vi "Synchronized Acquisition with Disk Streaming.vi"() -> ()   [LabVIEW 2021]
uses:
  <vilib>/userdefined/Silver/nirio_resource_slv.ctl
  Digitizer Control Class/Public/TClk API Control Enable.ctl
  Digitizer Control Class/Digitizer Control.lvclass
  Disk Streaming Class/Disk Streaming.lvclass
  Disk Streaming Class/Public/IO mode.ctl
  Digitizer Control Class/Public/Acq Start Trigger Type.ctl
panel:
  in  "PXIe?":bool=TRUE
  out "Samples Acquired":u64[](array[numeric])
  in  "Stop Button":bool
  in  "Tab Control":enum32{"Acquisition Preview", "I/O Performance"}(tab)
  out "Waveform Graph":waveform(dbl)[](graph)
  out "Power Spectrum":cluster{"f0":dbl, "df":dbl, "magnitude":dbl[]}[](graph) caption="Waveform Graph"
  out "Pending Disk Operations":u32[](graph)
  out "Host DMA buffer use":u64[](graph)
  out "Device Memory use":u64[][](graph)
  out "Device FIFO use":u64[][](graph)
  in  "# of blocks":u32=5
  in  "Preview # of samples":u32=10000
  in  "Reserve File Size?":bool
  in  "Disable Buffering?":bool=TRUE
  in  "I/O mode":T1(ring)=enum."Data Reference"
  in  "Block Duration (s)":dbl=0.01 format="%0.2p"
  in  "12-bit packing":bool
  out "Overflow":bool[](array[boolean])
  in  "Desired Sampling Rate":dbl=800000000.0 format="%0.2p"
  out "Actual IQ Rate":dbl format="%#_6p"
  in  "# of samples":i64=10000000
  in  "device and file selection":T3(array[cluster])
  # "Device / File Selection"
  # "Device"
  # "AI0 Destination File"
  # "AI1 Destination File"
  # "Acquisition Configuration"
  # "Acquisition Status"
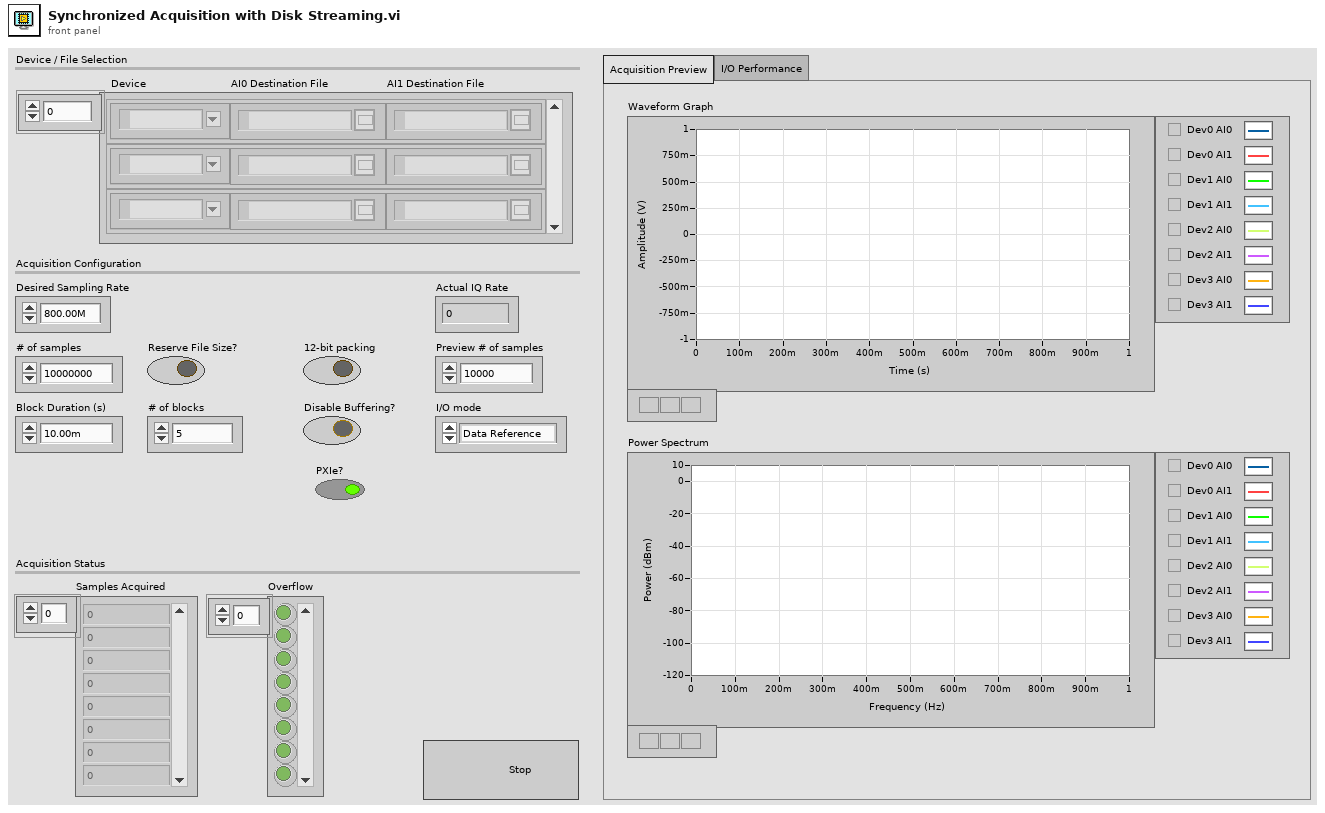
[diagram p1: front panel]
types:
  T1 = enum16{"Synchronous", "Asynchronous", "Data Reference"}
  T2 = typedef "nirio_resource_slv.ctl" = tag
  T3 = cluster{"RIO Device":T2, "AI0 File":path, "AI1 File":path}[]
  T4 = typedef "Digitizer Control.lvclass/TClk API Control Enable.ctl" = enum16{"None", "Acquisition"}
  T5 = typedef "Disk Streaming.lvclass/IO mode.ctl" = enum16{"Synchronous", "Asynchronous", "Data Reference"}
  T6 = cluster{"enabled":bool, "session":refnum<class "Digitizer Control.lvclass">, "channel index":i32, "sample count":i64, "disk streaming":refnum<class "Disk Streaming.lvclass">, "I/O mode":T5}
  T7 = typedef "Digitizer Control.lvclass/Acq Start Trigger Type.ctl" = enum16{"Immediate", "Analog", "Digital Edge", "Digital Level"}
  T8 = cluster{"enabled":bool, "session":refnum<class "Digitizer Control.lvclass">, "channel index":i32, "sample count":i64, "disk streaming":refnum<class "Disk Streaming.lvclass">, "I/O mode":T5}[]
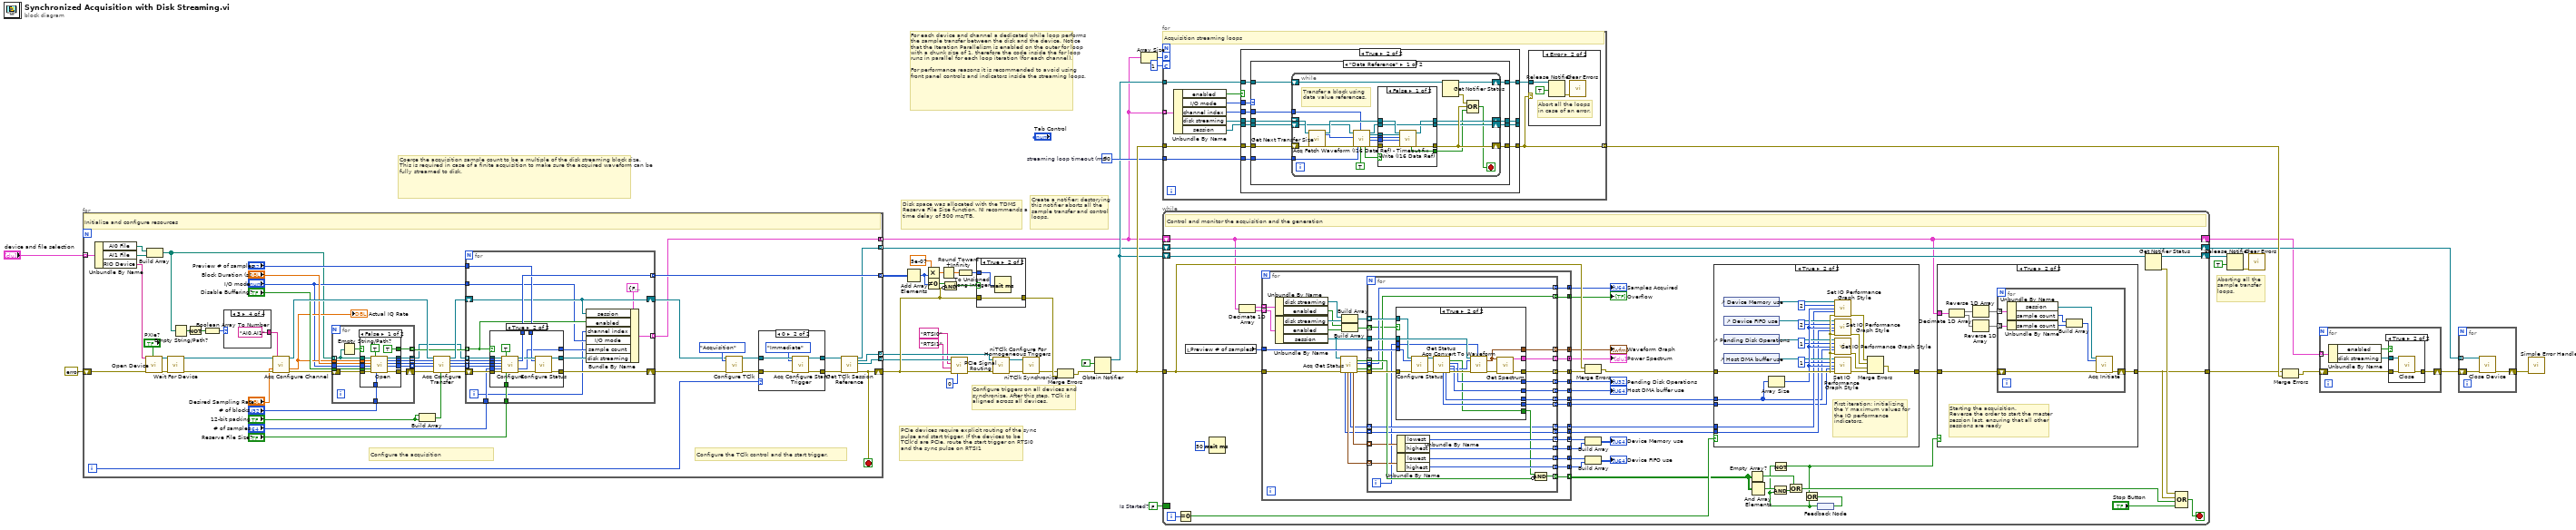
[diagram p0: block diagram]
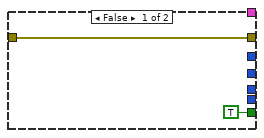
[diagram p5: hidden frame]
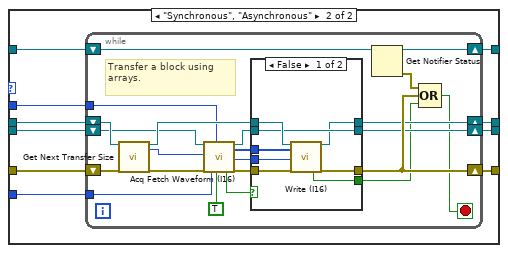
[diagram p9: hidden frame]
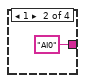
[diagram p13: hidden frame]
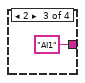
[diagram p14: hidden frame]
diagram:
  w5 = FALSE  # Is Started?
  w14 = 50  # streaming loop timeout (ms)
  # "Coerce the acquisition sample count to be a multiple of the disk streaming block size. This is required in case of a finite acquisition to make sure the acquired waveform can be fully streamed to disk."
  # "Aborting all the sample transfer loops."
  # "For each device and channel a dedicated while loop performs the sample transfer between the disk and the device. Notice that the Iteration Parallelism is enabled on the outer for loop with a chunk size of 1, therefore the code inside the for loop runs in parallel for each loop iteration (for each channel).\n\nFor performance reasons it is recommended to avoid using front panel controls and indicators inside the streaming loops."
  # "Create a notifier: destorying this notifier aborts all the sample transfer and control loops."
  # "Disk space was allocated with the TDMS Reserve File Size function. NI recommends a time delay of 500 ms/TB."
  # "PCIe devices require explicit routing of the sync pulse and start trigger. If the devices to be TClk'd are PCIe, route the start trigger on RTSI0 and the sync pulse on RTSI1"
  # "Configure triggers on all devices and\nsynchronize. After this step, TClk is\naligned across all devices."
  n1 = for {
    shift-right: [w48] -> w38
    shift-left: errorcluster {"status"=FALSE, "code"=0, "source"=""} ("error out") -> [w93]
    tunnel: "device and file selection" -> [w87] mode=indexing
    tunnel: [w89] -> w34 mode=indexing
    tunnel: [w88] -> w31 mode=indexing
    tunnel: [w90] -> w4 mode=indexing
    tunnel: [w49] -> w3 mode=concatenating
    tunnel: [w94] -> w27 mode=indexing
    i -> [w83]
    stop <- w48 stop-if-true
    # "Configure the acquisition"
    # "Configure the TClk control and the start trigger."
    # "Initialize and configure resources"
    n2 = Unbundle By Name(w87) -> ("AI0 File"=w66:path, "AI1 File"=w65:path, "RIO Device"=w86:T2)
    n3 = call "Open Device.vi"("resource name"=w86, "error in (no error)"=w93, "PXIe?"="PXIe?") -> ("session out"=w91:refnum<class "Digitizer Control.lvclass">, "error out"=w92:errorcluster)  [unwired: 15 in]
    n4 = Build Array(w66, w65) -> (w47:path[])
    n5 = call "Wait For Device.vi"("session in"=w91, "error in (no error)"=w92) -> ("session out"=w84:refnum<class "Digitizer Control.lvclass">, "error out"=w85:errorcluster)  [unwired: 15 in, 1 out]
    n6 = Empty String/Path?(string/path=w47) -> (empty?=w46:bool[])
    n7 = Not(x=w46) -> (.not. x?=w43:bool[])
    n8 = Boolean Array To Number(Boolean array=w43) -> (number=w45:u32)
    n9 = case shown="3" w45 {
      tunnel: [_ "AI0" ("AI channel") "AI1" ("AI channel") "AI0,AI1" ("AI channel")] -> w44
      frame Default {
      }
      frame 1 {
      }
      frame 2 {
      }
      frame 3 {
      }
    }
    n10 = call "Acq Configure Channel.vi"("session in"=w84, "sampling rate (SPS)"="Desired Sampling Rate", "error in (no error)"=w85, "AI channel"=w44) -> ("session out"=w79:refnum<class "Digitizer Control.lvclass">, "actual sampling rate (SPS)"=w68:dbl, "error out"=w80:errorcluster)  [unwired: 9 in, 4 out]
    "Actual IQ Rate" <- w68
    n11 = for {
      tunnel: [w151] -> w50 mode=indexing
      tunnel: "Block Duration (s)" -> [w150]
      tunnel: "Disable Buffering?" -> [w149]
      tunnel: "I/O mode" -> [w148]
      tunnel: "# of blocks" -> [w147]
      tunnel: w68 -> [w146]
      shift-right: [w153] -> w82
      shift-left: w80 -> [w152]
      tunnel: w47 -> [w145] mode=indexing
      tunnel: [w143] -> w52 mode=indexing
      tunnel: [w142] -> w64 mode=indexing
      tunnel: [w141] -> w63 mode=indexing
      tunnel: [w140] -> w62 mode=indexing
      n12 = Empty String/Path?(string/path=w145) -> (empty?=w144:bool)
      n13 = case shown="False" w144 {
        tunnel: [w167 w168] -> w153
        tunnel: w152 -> [w166 w168]
        tunnel: [w165 _] -> w151
        tunnel: w150 -> [w163 _]
        tunnel: w149 -> [w162 _]
        tunnel: w148 -> [w161 _]
        tunnel: w147 -> [w160 _]
        tunnel: w146 -> [w159 _]
        tunnel: w145 -> [w158 _]
        tunnel: [TRUE _] -> w143
        tunnel: [w156 _] -> w142
        tunnel: [w155 _] -> w141
        tunnel: [w154 _] -> w140
        frame False {
          n14 = call "Open.vi"("file path"=w158, "sample rate (SPS)"=w159, "block duration (s) (0.01)"=w163, "I/O mode (Data Reference)"=w161, "disable buffering? (T)"=w162, "error in (no error)"=w166, "disk read (F) / write (T)"=TRUE, "# of blocks (5)"=w160) -> ("disk streaming out"=w165:refnum<class "Disk Streaming.lvclass">, "host DMA buffer size (samples)"=w156:u32, "host DMA buffer num of blocks"=w155:u32, "host DMA buffer block size divisor (bytes)"=w154:u32, "error out"=w167:errorcluster)  [unwired: 7 in]
        }
        frame True {
        }
      }
    }
    n15 = Build Array("12-bit packing", "12-bit packing") -> (w67:bool[])
    n16 = call "Acq Configure Transfer.vi"("session in"=w79, "host DMA buffer size (samples)"=w64, "host DMA buffer num of blocks"=w63, "host DMA buffer block size divisor (bytes)"=w62, "error in (no error)"=w82, "enable bit packing (F)"=w67) -> ("session out"=w54:refnum<class "Digitizer Control.lvclass">, "actual host DMA buffer size (samples)"=w78:u32[], "actual host DMA buffer size (elements)"=w77:u32[], "transfer quantum size (samples)"=w76:u64[], "error out"=w81:errorcluster)  [unwired: 7 in, 2 out]
    n17 = for {
      tunnel: [w115] -> w94 mode=indexing
      tunnel: w78 -> [w113] mode=indexing
      tunnel: w77 -> [w112] mode=indexing
      tunnel: w76 -> [w111] mode=indexing
      tunnel: "Preview # of samples" -> [w110]
      tunnel: "Reserve File Size?" -> [w109]
      shift-right: [w108] -> w55
      shift-left: w81 -> [w114]
      tunnel: "# of samples" -> [w101]
      shift-right: [w105] -> w51
      shift-left: w54 -> [w105]
      tunnel: "I/O mode" -> [w102]
      tunnel: w52 -> [w104] mode=indexing
      tunnel: w50 -> [w107] mode=indexing
      tunnel: [w100] -> w49 mode=indexing
      i -> [w98]
      n18 = case shown="True" w104 {
        tunnel: [_ w132] -> w115
        tunnel: w114 -> [w116 w131]
        tunnel: [w117 w129] -> w106
        tunnel: w107 -> [w117 w127]
        tunnel: w113 -> [_ w126]
        tunnel: w112 -> [_ w125]
        tunnel: w111 -> [_ w124]
        tunnel: w110 -> [_ w123]
        tunnel: w101 -> [_ w122]
        tunnel: w109 -> [_ w121]
        tunnel: [_ w120] -> w103
        tunnel: [w116 w118] -> w108
        frame False {
        }
        frame True {
          n19 = call "Configure.vi"("disk streaming in"=w127, "actual host DMA buffer size (samples)"=w126, "actual host DMA buffer size (elements)"=w125, "transfer quantum size (samples)"=w124, "sample count (-1)"=w122, "error in (no error)"=w131, "coerce sample count? (T)"=TRUE, "reserve file size (F)"=w121) -> ("disk streaming out"=w128:refnum<class "Disk Streaming.lvclass">, "file allocation size (bytes)"=w132:u64, "sample count out"=w120:i64, "error out"=w130:errorcluster)  [unwired: 6 in, 2 out]
          n20 = call "Configure Status.vi"("disk streaming in"=w128, "preview size (samples)"=w123, "error in (no error)"=w130) -> ("disk streaming out"=w129:refnum<class "Disk Streaming.lvclass">, "error out"=w118:errorcluster)  [unwired: 15 in]
        }
      }
      n21 = Bundle By Name(cluster=T6 {"enabled"=FALSE, "session"=refnum, "channel index"=0, "sample count"=0, "disk streaming"=refnum, "I/O mode"=enum."Synchronous"}, "session"=w105, "enabled"=w104, "channel index"=w98, "I/O mode"=w102, "sample count"=w103, "disk streaming"=w106) -> (w100:T6)
    }
    n22 = call "Configure TClk.vi"("session in"=w51, "TClk API Control Enable"=TClk_API_Control_Enable."Acquisition", "error in (no error)"=w55) -> ("session out"=w58:refnum<class "Digitizer Control.lvclass">, "error out"=w59:errorcluster)  [unwired: 15 in]
    n23 = case shown="0" w83 {
      tunnel: w59 -> [w133 w139]
      tunnel: w58 -> [w134 w138]
      tunnel: [w133 w136] -> w57
      tunnel: [w134 w135] -> w56
      frame Default {
      }
      frame 0 {
        n24 = call "Acq Configure Start Trigger.vi"("session in"=w138, "trigger type (Immediate)"=Acq_Start_Trigger_Type."Immediate" ("trigger type"), "error in (no error)"=w139) -> ("session out"=w135:refnum<class "Digitizer Control.lvclass">, "error out"=w136:errorcluster)  [unwired: 15 in]
      }
    }
    n25 = call "Get TClk Session Reference.vi"("session in"=w56, "error in (no error)"=w57) -> ("session out"=w90:refnum<class "Digitizer Control.lvclass">, "tclk session reference"=w88:refnum<k20>, "fpga reference"=w89:refnum<k20>, "error out"=w48:errorcluster)  [unwired: 14 in]
  }
  n26 = Add Array Elements(numeric array=w27) -> (sum=w23:u64)
  n27 = Multiply(x=5e-07, y=w23) -> (x*y=w21:dbl)
  n28 = Not Equal To 0?(x=w23) -> (x != 0?=w26:bool)
  n29 = Round Toward +Infinity(x=w21) -> (ceil(x): smallest int >= x=w20:dbl)
  n30 = Compound Arithmetic op=AND(w26, invert w38) -> (w25:bool)
  n31 = call "PCIe Signal Routing.vi"("trigger master index"=0, "error in (no error)"=w38, "sync pulse rtsi line"="RTSI1", "start trigger rtsi line"="RTSI0", "fpga interfaces in"=w34) -> ("error out"=w32:errorcluster)  [unwired: 5 in, 1 out]
  n32 = To Unsigned Long Integer(number=w20) -> (unsigned 32bit integer=w19:u32)
  n33 = case shown="True" w25 {
    tunnel: w38 -> [w169 w171]
    tunnel: [w169 w171] -> w39
    tunnel: w19 -> [_ w170]
    frame False {
    }
    frame True {
      n34 = Wait (ms)(milliseconds to wait=w170) -> ()  [unwired: 1 out]
    }
  }
  n35 = call <instrlib>:"niTClk Configure For Homogeneous Triggers.vi"("error in (no error)"=w32, "sessions"=w31) -> ("error out"=w37:errorcluster, "sessions out"=w36:refnum<k20>[])  [unwired: 8 in]
  n36 = call <instrlib>:"niTClk Synchronize.vi"("error in (no error)"=w37, "sessions"=w36) -> ("error out"=w24:errorcluster)  [unwired: 8 in, 1 out]
  n37 = Merge Errors(w24, w39) -> (w18:errorcluster)
  n38 = Obtain Notifier(notification data type=FALSE, error in (no error)=w18) -> (notifier out=w13:refnum<notifier>, error out=w41:errorcluster)  [unwired: 2 in, 1 out]
  n39 = Array Size(array=w3) -> (size(s)=w16:i32)
  n40 = for {
    workers-P: w16 -> [_]
    chunk-C: 1 -> [_]
    tunnel: w3 -> [w182] mode=indexing
    tunnel: w41 -> [w177]
    tunnel: w14 -> [w176]
    tunnel: w13 -> [w175]
    tunnel: [w174] -> w40 mode=indexing
    # "Acquisition streaming loops"
    n41 = Unbundle By Name(w182) -> ("enabled"=w181:bool, "I/O mode"=w180:T5, "channel index"=w172:i32, "disk streaming"=w179:refnum<class "Disk Streaming.lvclass">, "session"=w178:refnum<class "Digitizer Control.lvclass">)
    n42 = case shown="True" w181 {
      tunnel: w180 -> [_ w200]
      tunnel: w179 -> [w187 w197]
      tunnel: w178 -> [w188 w198]
      tunnel: w177 -> [w189 w199]
      tunnel: w176 -> [_ w196]
      tunnel: w175 -> [w186 w195]
      tunnel: [w186 w194] -> w173
      tunnel: [w187 w193] -> _
      tunnel: [w188 w192] -> _
      tunnel: [w189 w191] -> w174
      tunnel: w172 -> [_ w190]
      frame False {
        # "Acquisition is not enabled for this device and channel."
      }
      frame True {
        n43 = case shown="\"Data Reference\"" w200 {
          tunnel: w199 -> [w210 w255]
          tunnel: w198 -> [w209 w254]
          tunnel: w197 -> [w208 w253]
          tunnel: w196 -> [w207 w252]
          tunnel: w195 -> [w206 w251]
          tunnel: [w205 w250] -> w194
          tunnel: [w204 w249] -> w193
          tunnel: [w203 w248] -> w192
          tunnel: [w202 w247] -> w191
          tunnel: w190 -> [w201 w246]
          frame "Data Reference" {
            n44 = while {
              tunnel: w207 -> [w227]
              shift-right: [w223] -> w205
              shift-left: w206 -> [w224]
              shift-right: [w225] -> w204
              shift-left: w208 -> [w231]
              shift-right: [w226] -> w203
              shift-left: w209 -> [w228]
              shift-right: [w233] -> w202
              shift-left: w210 -> [w232]
              tunnel: w201 -> [w211]
              stop <- w213 stop-if-true
              # "Transfer a block using data value references."
              n45 = call "Get Next Transfer Size.vi"("disk streaming in"=w231, "error in (no error)"=w232) -> ("disk streaming out"=w230:refnum<class "Disk Streaming.lvclass">, "elements to transfer"=w214:u32, "error out"=w229:errorcluster)  [unwired: 15 in]
              n46 = call "Acq Fetch Waveform (I16 Data Ref) - Timeout fix.vi"("session in"=w228, "elements to read"=w214, "error in (no error)"=w229, "timeout (ms)"=w227, "channel index"=w211, "clear time out error? (F)"=TRUE) -> ("timed out?"=w216:bool, "session out"=w217:refnum<class "Digitizer Control.lvclass">, "sample data"=w220:refnum<data-value>, "elements in region"=w219:u32, "elements remaining"=w218:u32, "error out"=w221:errorcluster)  [unwired: 8 in]
              n47 = case shown="False" w216 {
                tunnel: w230 -> [w242 w245]
                tunnel: w221 -> [w241 w243]
                tunnel: w220 -> [w240 _]
                tunnel: w219 -> [w239 _]
                tunnel: w218 -> [w238 _]
                tunnel: w217 -> [w237 w244]
                tunnel: [w237 w244] -> w226
                tunnel: [w236 _] -> w212
                tunnel: [w235 w243] -> w233
                tunnel: [w234 w245] -> w225
                frame False {
                  n48 = call "Write (I16 Data Ref).vi"("disk streaming in"=w242, "sample data"=w240, "elements in region"=w239, "elements remaining"=w238, "error in (no error)"=w241) -> ("finished"=w236:bool, "disk streaming out"=w234:refnum<class "Disk Streaming.lvclass">, "error out"=w235:errorcluster)  [unwired: 11 in, 1 out]
                }
                frame True {
                  # "Fetch timed out."
                }
              }
              n49 = Get Notifier Status(notifier=w224) -> (notifier out=w223:refnum<notifier>, error out=w215:errorcluster)  [unwired: 1 in, 3 out]
              n50 = Compound Arithmetic op=OR(w215, w233, w212) -> (w213:bool)
            }
          }
          frame "Synchronous", "Asynchronous" {
            n51 = while {
              tunnel: w252 -> [w271]
              shift-right: [w267] -> w250
              shift-left: w251 -> [w268]
              shift-right: [w269] -> w249
              shift-left: w253 -> [w275]
              shift-right: [w270] -> w248
              shift-left: w254 -> [w272]
              shift-right: [w277] -> w247
              shift-left: w255 -> [w276]
              tunnel: w246 -> [w256]
              stop <- w258 stop-if-true
              # "Transfer a block using arrays."
              n52 = call "Get Next Transfer Size.vi"("disk streaming in"=w275, "error in (no error)"=w276) -> ("disk streaming out"=w274:refnum<class "Disk Streaming.lvclass">, "elements to transfer"=w259:u32, "error out"=w273:errorcluster)  [unwired: 15 in]
              n53 = call "Acq Fetch Waveform (I16).vi"("session in"=w272, "elements to read"=w259, "error in (no error)"=w273, "timeout (ms)"=w271, "channel index"=w256, "clear time out error? (F)"=TRUE) -> ("timed out?"=w261:bool, "session out"=w262:refnum<class "Digitizer Control.lvclass">, "sample data"=w264:i16[], "elements remaining"=w263:u32, "error out"=w265:errorcluster)  [unwired: 9 in]
              n54 = case shown="False" w261 {
                tunnel: w274 -> [w285 w288]
                tunnel: w265 -> [w284 w286]
                tunnel: w264 -> [w283 _]
                tunnel: w263 -> [w282 _]
                tunnel: w262 -> [w281 w287]
                tunnel: [w281 w287] -> w270
                tunnel: [w280 _] -> w257
                tunnel: [w279 w286] -> w277
                tunnel: [w278 w288] -> w269
                frame False {
                  n55 = call "Write (I16).vi"("disk streaming in"=w285, "sample data"=w283, "elements remaining"=w282, "error in (no error)"=w284) -> ("finished"=w280:bool, "disk streaming out"=w278:refnum<class "Disk Streaming.lvclass">, "error out"=w279:errorcluster)  [unwired: 12 in, 1 out]
                }
                frame True {
                  # "Fetch timed out."
                }
              }
              n56 = Get Notifier Status(notifier=w268) -> (notifier out=w267:refnum<notifier>, error out=w260:errorcluster)  [unwired: 1 in, 3 out]
              n57 = Compound Arithmetic op=OR(w260, w277, w257) -> (w258:bool)
            }
          }
        }
      }
    }
    n58 = case shown="Error" w174 {
      tunnel: w173 -> [_ w185]
      frame No Error {
      }
      frame Error {
        # "Abort all the loops in case of an error."
        n59 = Release Notifier(notifier=w185, force destroy? (F)=TRUE) -> (error out=w183:errorcluster)  [unwired: 1 in, 2 out]
        n60 = call <vilib>:"Clear Errors.vi"("error in (no error)"=w183) -> ()  [unwired: 5 in, 2 out]
      }
    }
  }
  n61 = while {
    tunnel: w41 -> [w330]
    tunnel: [w309] -> w9
    shift-right: [w315] -> w10
    shift-left: w13 -> [w328]
    border: w5 -> [_]
    shift-right: [w311] -> w2
    shift-left: w4 -> [w311]
    shift-right: [w304] -> w1
    shift-left: w3 -> [w304]
    i -> [w290]
    stop <- w289 stop-if-true
    # "Control and monitor the acquisition and the generation"
    n62 = Equal To 0?(x=w290) -> (x = 0?=w325:bool)
    n63 = local read "Preview # of samples"() -> (w329:u32)
    n64 = Wait (ms)(milliseconds to wait=u32 50) -> ()  [unwired: 1 out]
    n65 = Decimate 1D Array(w304) -> (w303:T8, w302:T8)
    n66 = for {
      tunnel: w303 -> [w400] mode=indexing
      tunnel: w330 -> [w401]
      tunnel: w329 -> [w399]
      tunnel: [w375] -> w299 mode=concatenating
      tunnel: [w373] -> w300 mode=concatenating
      tunnel: [w398] -> w318 mode=indexing
      tunnel: [w397] -> w306 mode=concatenating
      tunnel: [w396] -> w305 mode=concatenating
      tunnel: [w395] -> w322 mode=concatenating
      tunnel: [w394] -> w321 mode=concatenating
      tunnel: [w393] -> w298 mode=concatenating
      tunnel: [w371] -> w327 mode=concatenating
      tunnel: [w392] -> w297 mode=concatenating
      tunnel: [w391] -> w296 mode=concatenating
      tunnel: [w390] -> w295 mode=concatenating
      tunnel: [w389] -> w293 mode=concatenating
      tunnel: [w388] -> w292 mode=concatenating
      tunnel: [w379] -> w324 mode=concatenating
      tunnel: [w377] -> w323 mode=concatenating
      tunnel: w302 -> [w387] mode=indexing
      n67 = Unbundle By Name(w400) -> ("disk streaming"=w370:refnum<class "Disk Streaming.lvclass">, "enabled"=w368:bool)
      n68 = Unbundle By Name(w387) -> ("disk streaming"=w369:refnum<class "Disk Streaming.lvclass">, "enabled"=w367:bool, "session"=w386:refnum<class "Digitizer Control.lvclass">)
      n69 = call "Acq Get Status.vi"("session in"=w386, "error in (no error)"=w401) -> ("FIFO size"=w378:u64[], "FIFO utilization"=w383:cluster{"lowest":u64, "highest":u64}[], "memory size"=w380:u64[], "memory utilization"=w384:cluster{"lowest":u64, "highest":u64}[], "acquiring"=w385:bool[], "samples acquired"=w376:u64[], "overflow"=w374:bool[], "error out"=w372:errorcluster)  [unwired: 8 in, 2 out]
      n70 = Build Array(w370, w369) -> (w382:refnum<class "Disk Streaming.lvclass">[])
      n71 = Build Array(w368, w367) -> (w381:bool[])
      n72 = for {
        tunnel: w399 -> [w425]
        tunnel: [w424] -> w398 mode=indexing
        tunnel: [w423] -> w397 mode=indexing
        tunnel: [w422] -> w396 mode=indexing
        tunnel: [w421] -> w395 mode=indexing
        tunnel: [w420] -> w394 mode=indexing
        tunnel: [w419] -> w393 mode=indexing
        tunnel: [w418] -> w392 mode=indexing
        tunnel: [w417] -> w391 mode=indexing
        tunnel: [w416] -> w390 mode=indexing
        tunnel: [w415] -> w389 mode=indexing
        tunnel: [w414] -> w388 mode=indexing
        tunnel: w386 -> [w413]
        tunnel: w385 -> [w412] mode=indexing
        tunnel: w384 -> [w411] mode=indexing
        tunnel: w383 -> [w410] mode=indexing
        tunnel: w382 -> [w408] mode=indexing
        tunnel: w381 -> [w403] mode=indexing
        tunnel: w380 -> [w407] mode=indexing
        tunnel: [w407] -> w379 mode=indexing
        tunnel: w378 -> [w406] mode=indexing
        tunnel: [w406] -> w377 mode=indexing
        tunnel: w376 -> [w405] mode=indexing
        tunnel: [w405] -> w375 mode=indexing
        tunnel: w374 -> [w404] mode=indexing
        tunnel: [w404] -> w373 mode=indexing
        tunnel: w372 -> [w427]
        tunnel: [w426] -> w371 mode=indexing
        i -> [w402]
        n73 = case shown="True" w403 {
          tunnel: w427 -> [w429 w444]
          tunnel: [w429 w443] -> w426
          tunnel: w425 -> [_ w442]
          tunnel: [_ w441] -> w423
          tunnel: [_ w440] -> w422
          tunnel: [_ w439] -> w421
          tunnel: [_ w438] -> w420
          tunnel: [_ w437] -> w419
          tunnel: [_ w436] -> w418
          tunnel: w413 -> [_ w435]
          tunnel: [TRUE ("finished") w432] -> w409
          tunnel: w408 -> [_ w431]
          tunnel: w402 -> [_ w430]
          frame False {
          }
          frame True {
            n74 = call "Configure Status.vi"("disk streaming in"=w431, "preview size (samples)"=w442, "error in (no error)"=w444) -> ("disk streaming out"=w433:refnum<class "Disk Streaming.lvclass">, "error out"=w447:errorcluster)  [unwired: 15 in]
            n75 = call "Get Status.vi"("disk streaming in"=w433, "error in (no error)"=w447) -> ("Host DMA buffer size (bytes)"=w438:u64, "Disk maximum async operations"=w439:u32, "finished"=w432:bool, "Disk pending async operations"=w441:u32, "Host DMA buffer utilization (bytes)"=w440:u64, "preview data"=w434:i16[], "error out"=w446:errorcluster)  [unwired: 10 in, 1 out]
            n76 = call "Acq Convert To Waveform.vi"("session in"=w435, "sample data"=w434, "error in (no error)"=w446, "channel index"=w430) -> ("waveform (V)"=w437:waveform(dbl), "error out"=w445:errorcluster)  [unwired: 13 in, 1 out]
            n77 = call "Get Spectrum.vi"("waveform (V)"=w437, "error in (no error)"=w445) -> ("power spectrum (dBm)"=w436:cluster{"f0":dbl, "df":dbl, "magnitude":dbl[]}, "error out"=w443:errorcluster)  [unwired: 12 in]
          }
        }
        n78 = Unbundle By Name(w411) -> ("lowest"=w417:u64, "highest"=w416:u64)
        n79 = Unbundle By Name(w410) -> ("lowest"=w415:u64, "highest"=w414:u64)
        n80 = Compound Arithmetic op=AND(w409, invert w412) -> (w424:bool)
      }
    }
    "Waveform Graph" <- w298
    "Samples Acquired" <- w299
    "Overflow" <- w300
    "Power Spectrum" <- w297
    "Pending Disk Operations" <- w306
    "Host DMA buffer use" <- w305
    n81 = Merge Errors(w330, w327) -> (w326:errorcluster)
    n82 = Build Array(w296, w295) -> (→"Device Memory use":u64[][])
    n83 = Build Array(w293, w292) -> (→"Device FIFO use":u64[][])
    n84 = case shown="True" w325 {
      tunnel: w326 -> [w347 w366]
      tunnel: w324 -> [_ w355]
      tunnel: w323 -> [_ w354]
      tunnel: w322 -> [_ w349]
      tunnel: w321 -> [_ w352]
      tunnel: [w347 w348] -> w310
      frame False {
      }
      frame True {
        # "First iteration: initializing the Y maximum values for the IO performance indicators."
        n85 = control-ref of="Device Memory use"() -> (w364:refnum<vi>)
        n86 = control-ref of="Device FIFO use"() -> (w362:refnum<vi>)
        n87 = control-ref of="Pending Disk Operations"() -> (w357:refnum<vi>)
        n88 = control-ref of="Host DMA buffer use"() -> (w356:refnum<vi>)
        n89 = Array Size(array=w349) -> (size(s)=w365:i32)
        n90 = call "Set IO Performance Graph Style.vi"("Waveform Graph Refnum"=w364, "# of plots (1)"=2, "# of devices (1)"=w365, "Y maximum (1)"=w355, "error in (no error)"=w366) -> ("error out"=w360:errorcluster)  [unwired: 10 in]
        n91 = call "Set IO Performance Graph Style.vi"("Waveform Graph Refnum"=w362, "# of plots (1)"=2, "# of devices (1)"=w365, "Y maximum (1)"=w354, "error in (no error)"=w366) -> ("error out"=w353:errorcluster)  [unwired: 10 in]
        n92 = call "Set IO Performance Graph Style.vi"("Waveform Graph Refnum"=w357, "# of plots (1)"=1, "# of devices (1)"=w365, "Y maximum (1)"=w349, "error in (no error)"=w366) -> ("error out"=w350:errorcluster)  [unwired: 10 in]
        n93 = call "Set IO Performance Graph Style.vi"("Waveform Graph Refnum"=w356, "# of plots (1)"=1, "# of devices (1)"=w365, "Y maximum (1)"=w352, "error in (no error)"=w366) -> ("error out"=w351:errorcluster)  [unwired: 10 in]
        n94 = Merge Errors(w360, w353, w350, w351) -> (w348:errorcluster)
      }
    }
    n95 = Empty Array?(array=w318) -> (empty?=w317:bool)
    n96 = And Array Elements(Boolean array=w318) -> (logical AND=w314:bool)
    n97 = feedback #1() -> (w308:bool)
    n98 = And(x=w314, y=w308) -> (x .and. y?=w313:bool)
    n99 = Not(x=w308) -> (.not. x?=w307:bool)
    n100 = Or(x=w317, y=w313) -> (x .or. y?=w319:bool)
    n101 = Or(x=w307, y=w308) -> (x .or. y?=w312:bool)
    n102 = feedback-in #1(w312) -> ()
    n103 = case shown="True" w307 {
      tunnel: w304 -> [_ w335]
      tunnel: w310 -> [w331 w337]
      tunnel: [w331 w336] -> w309
      frame False {
      }
      frame True {
        # "Starting the acquisition.\nReverse the order to start the master session last, ensuring that all other sessions are ready"
        n104 = Decimate 1D Array(w335) -> (w334:T8, w333:T8)
        n105 = Reverse 1D Array(array=w334) -> (reversed array=w338:T8)
        n106 = Reverse 1D Array(array=w333) -> (reversed array=w332:T8)
        n107 = for {
          tunnel: w338 -> [w346] mode=indexing
          shift-right: [w344] -> w336
          shift-left: w337 -> [w343]
          tunnel: w332 -> [w342] mode=indexing
          n108 = Unbundle By Name(w346) -> ("session"=w345:refnum<class "Digitizer Control.lvclass">, "sample count"=w341:i64)
          n109 = Unbundle By Name(w342) -> ("sample count"=w340:i64)
          n110 = Build Array(w341, w340) -> (w339:i64[])
          n111 = call "Acq Initiate.vi"("session in"=w345, "sample count (-1)"=w339, "error in (no error)"=w343) -> ("error out"=w344:errorcluster)  [unwired: 10 in, 6 out]
        }
      }
    }
    n112 = Get Notifier Status(notifier=w328) -> (notifier out=w315:refnum<notifier>, error out=w316:errorcluster)  [unwired: 1 in, 3 out]
    n113 = Compound Arithmetic op=OR(w316, w309, w319, "Stop Button") -> (w289:bool)
  }
  n114 = Release Notifier(notifier=w10, force destroy? (F)=TRUE) -> (error out=w11:errorcluster)  [unwired: 1 in, 2 out]
  n115 = call <vilib>:"Clear Errors.vi"("error in (no error)"=w11) -> ()  [unwired: 5 in, 2 out]
  n116 = Merge Errors(w9, w40) -> (w8:errorcluster)
  n117 = for {
    shift-right: [w448] -> w7
    shift-left: w8 -> [w451]
    tunnel: w1 -> [w452] mode=indexing
    n118 = Unbundle By Name(w452) -> ("enabled"=w450:bool, "disk streaming"=w449:refnum<class "Disk Streaming.lvclass">)
    n119 = case shown="True" w450 {
      tunnel: w451 -> [w453 w456]
      tunnel: w449 -> [_ w455]
      tunnel: [w453 w454] -> w448
      frame False {
      }
      frame True {
        n120 = call "Close.vi"("disk streaming in"=w455, "error in (no error)"=w456) -> ("error out"=w454:errorcluster)  [unwired: 17 in]
      }
    }
  }
  n121 = for {
    tunnel: w2 -> [w457] mode=indexing
    shift-right: [w458] -> w6
    shift-left: w7 -> [w459]
    n122 = call "Close Device.vi"("session in"=w457, "error in (no error)"=w459) -> ("error out"=w458:errorcluster)  [unwired: 17 in]
  }
  n123 = call <vilib>:"Simple Error Handler.vi"("error in (no error)"=w6) -> ()  [unwired: 4 in, 5 out]
